vi "Tbl_Remove (SubVI).vi"(11 "Table in":refnum<vi>) -> ()   [LabVIEW 2017]
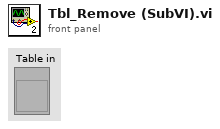
[diagram p1: front panel]
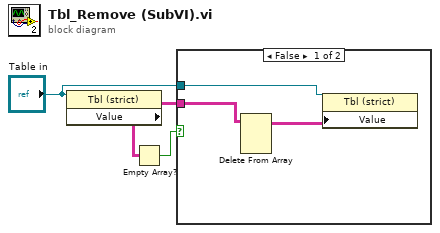
[diagram p0: block diagram]
diagram:
  n1 = property class="Tbl (strict)"(reference="Table in") -> ("Value"=w3:string[][])  [unwired: 1 in, 2 out]
  n2 = Empty Array?(array=w3) -> (empty?=w2:bool)
  n3 = case shown="False" w2 {
    tunnel: w3 -> [w6 _]
    tunnel: "Table in" -> [w4 _]
    frame False {
      n4 = Delete From Array(array=w6) -> (array with subset deleted=w5:string[][])  [unwired: 3 in, 1 out]
      n5 = property class="Tbl (strict)"(reference=w4, "Value"=w5) -> ()  [unwired: 1 in, 2 out]
    }
    frame True {
    }
  }
